vi "Write DWA Information.vi"(10 "DWA Information":T1={"Min"=29.75, "Max"=50.0, "Step"=0.75, "Default"=0.75}, 11 "Toggle 7.1 in":refnum<class "Toggle 7.1.lvclass">) -> (3 "Toggle 7.1 out":refnum<class "Toggle 7.1.lvclass">)   [LabVIEW 2020, in "Toggle 7.1.lvclass"]
uses:
  Toggle 7.1.lvclass
  Controls/Charge Pump Information cluster.ctl
  Toggle 7.1.lvclass/Toggle 7.1.ctl
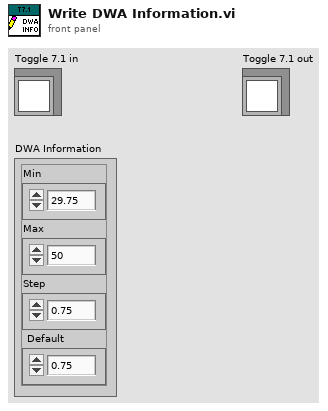
[diagram p1: front panel]
types:
  T1 = typedef "Toggle 7.1.lvclass/Charge Pump Information cluster.ctl" = cluster{"Min":dbl, "Max":dbl, "Step":dbl, "Default":dbl}
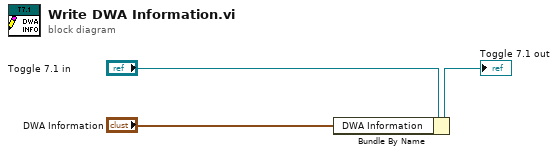
[diagram p0: block diagram]
diagram:
  n1 = Bundle By Name(cluster="Toggle 7.1 in", "DWA Information"="DWA Information") -> (→"Toggle 7.1 out":refnum<class "Toggle 7.1.lvclass">)
